vi "motor speed.vi"(0 "IN_A":refnum<k21>="ConnectorA/DIO2", 1 "IN_B":refnum<k21>="ConnectorA/DIO0", 3 "PWM":refnum<k21>="ConnectorA/DIO8", 4 "speed":i64, 5 "periode":i64, 6 "enable divider":bool, 7 "divider":fxp<+,4,4>, 9 "brake":bool) -> ()   [LabVIEW 2019]
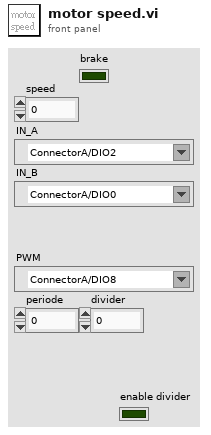
[diagram p1: front panel]
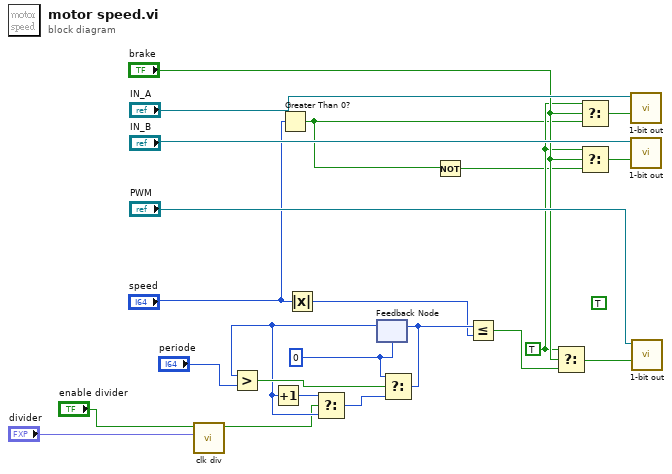
[diagram p0: block diagram]
diagram:
  w3 = TRUE ("t")
  (unwired) TRUE ("OUT")
  w23 = i64 0
  n1 = call "clk div.vi"("divider"="divider", "enable divider"="enable divider") -> ("f"=w15:bool)  [unwired: 9 in]
  n2 = Greater Than 0?(x="speed") -> (x > 0?=w1:bool)
  n3 = Absolute Value(x="speed") -> (abs(x)=w13:i64)
  n4 = feedback #1(w23) -> (w17:i64)
  n5 = Greater?(x=w17, y="periode") -> (0:w21:bool)
  n6 = Increment(x=w17) -> (x+1=w20:i64)
  n7 = Select(t=w20, s=w15, f=w17) -> (s? t:f=w19:i64)
  n8 = Select(t=w23, s=w21, f=w19) -> (s? t:f=w14:i64)
  n9 = feedback-in #1(w14) -> ()
  n10 = Not(x=w1) -> (.not. x?=w2:bool)
  n11 = Less Or Equal?(x=w14, y=w13) -> (x <= y?=w10:bool)
  n12 = Select(t=w3, s="brake", f=w10) -> (s? t:f=w11:bool)
  n13 = Select(t=w3, s="brake", f=w1) -> (s? t:f=w5:bool)
  n14 = Select(t=w3, s="brake", f=w2) -> (s? t:f=w6:bool)
  n15 = call "1-bit out.vi"("OUT"=w5, "DIO Refnum"="IN_A") -> ()  [unwired: 10 in]
  n16 = call "1-bit out.vi"("OUT"=w6, "DIO Refnum"="IN_B") -> ()  [unwired: 10 in]
  n17 = call "1-bit out.vi"("OUT"=w11, "DIO Refnum"="PWM") -> ()  [unwired: 10 in]
